vi "Get Data I16.vi"(8 "error in (no error)":errorcluster, 11 "Red Pitaya Digitizer in":refnum<class "Red Pitaya Digitizer.lvclass">) -> (0 "error out":errorcluster, 1 "Current read position":i32, 2 "Data out":i16[][](array[numeric]), 3 "Red Pitaya Digitizer out":refnum<class "Red Pitaya Digitizer.lvclass">, 4 "Finished":bool)   [LabVIEW 2016, in "Red Pitaya Digitizer.lvclass"]
uses:
  Red Pitaya Digitizer.lvclass
  C:/github/NHMFL_Core/Libraries/Instruments/Pulse Driver/Pulse Driver.lvclass
  Red Pitaya Digitizer.lvclass/Red Pitaya Digitizer.ctl
  Instruments/Pulse Driver/Pulse Driver.lvclass/Pulse Driver.ctl
  Read RP Instrument.vi
  Instruments/Pulse Driver/Read Pretrigger samples.vi
  Instruments/Pulse Driver/Read Samples per channel.vi
  Instruments/Pulse Driver/Read Current read position.vi
  Write RP Instrument.vi
  RP Core/RP Instrument/RP Instrument.lvclass
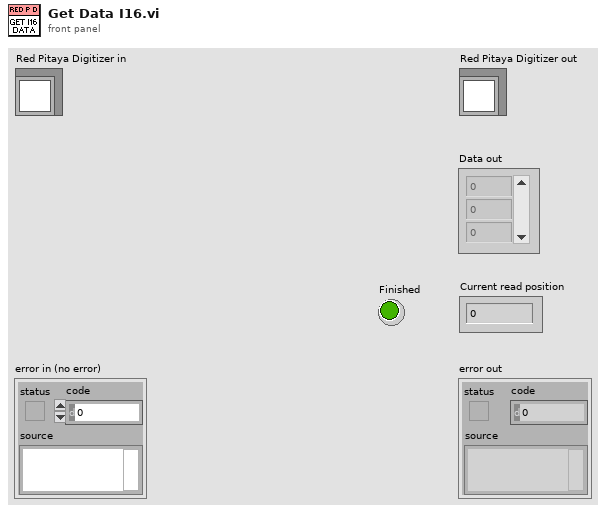
[diagram p1: front panel]
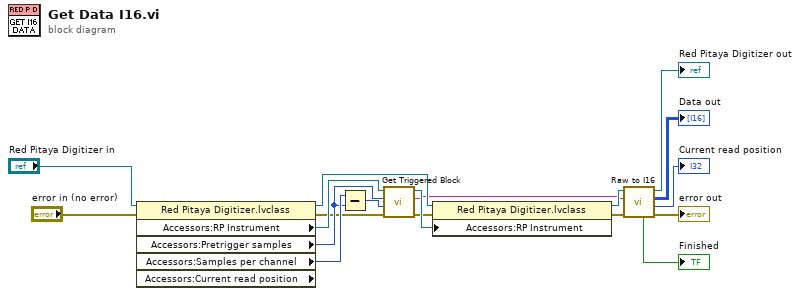
[diagram p0: block diagram]
diagram:
  n1 = property class="Red Pitaya Digitizer.lvclass" props=["Accessors:RP Instrument", "Accessors:Pretrigger samples", "Accessors:Samples per channel", "Accessors:Current read position"](reference="Red Pitaya Digitizer in", error in="error in (no error)") -> (reference out=w17:refnum<class "Red Pitaya Digitizer.lvclass">, error out=w11:errorcluster, "Accessors:RP Instrument"=w15:refnum<class "RP Instrument.lvclass">, "Accessors:Pretrigger samples"=w13:u32, "Accessors:Samples per channel"=w14:i32)  [unwired: 1 out]
  n2 = Subtract(x=w14, y=w13) -> (x-y=w12:u32)
  n3 = call-dynamic "Get Triggered Block.vi"("error in (no error)"=w11, "Post-trigger points"=w12, "Pre-trigger points"=w13, "RP Instrument in"=w15) -> ("error out"=w9:errorcluster, "Data out"=w1:string, "RP Instrument out"=w10:refnum<class "RP Instrument.lvclass">)  [unwired: 5 in]
  n4 = property class="Red Pitaya Digitizer.lvclass"(reference=w17, error in=w9, "Accessors:RP Instrument"=w10) -> (reference out=w8:refnum<class "Red Pitaya Digitizer.lvclass">, error out=w6:errorcluster)
  n5 = call-dynamic "Raw to I16.vi"("error in (no error)"=w6, "Raw data"=w1, "Red Pitaya Digitizer in"=w8) -> ("error out"=→"error out":errorcluster, "Current read position"=→"Current read position":i32, "Data out"=→"Data out":i16[][], "Red Pitaya Digitizer out"=→"Red Pitaya Digitizer out":refnum<class "Red Pitaya Digitizer.lvclass">, "Finished"=→"Finished":bool)  [unwired: 4 in]
